vi "Read Type.vi"(8 "error in (no error)":errorcluster, 11 "VoiceMeeterRemote in":refnum<class "VoiceMeeterRemote.lvclass">) -> (0 "error out":errorcluster, 3 "VoiceMeeterRemote out":refnum<class "VoiceMeeterRemote.lvclass">)   [LabVIEW 2020, in "VoiceMeeterRemote.lvlib" / "VoiceMeeterRemote.lvclass"]
uses:
  VoiceMeeterRemote.lvclass
  VoiceMeeterRemote.lvclass/VoiceMeeterRemote.ctl
  Voicemeeter Type.ctl
  VoiceMeeterRemote.lvlib
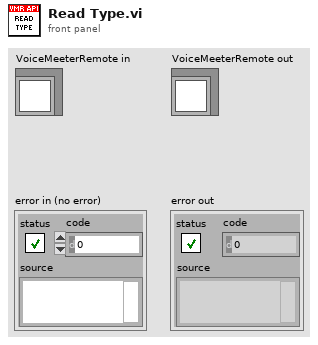
[diagram p1: front panel]
types:
  T1 = typedef "VoiceMeeterRemote.lvlib/Voicemeeter Type.ctl" = enum16{"Unknown", "Voicemeeter", "Banana", "Potato", "Potato x64"}
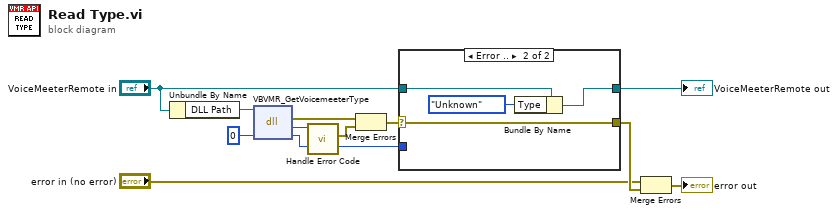
[diagram p0: block diagram]
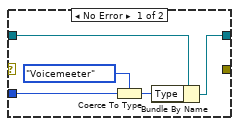
[diagram p2: hidden frame]
diagram:
  n1 = Unbundle By Name("VoiceMeeterRemote in") -> ("DLL Path"=w10:path)
  n2 = dll-call lib="C:/Program Files/National Instruments/LabVIEW 2022/user.lib/VoicemeeterRemote64/VoicemeeterRemote64.*" fn="VBVMR_GetVoicemeeterType"(path in=w10, "pType"=0) -> (error out=w7:errorcluster, "return type"=w8:i32, "pType"=w4:i32)  [unwired: 2 in, 1 out]
  n3 = call "Handle Error Code.vi"("Code"=w8) -> ("error out"=w6:errorcluster)  [unwired: 10 in]
  n4 = Merge Errors(w7, w6) -> (w5:errorcluster)
  n5 = case shown="Error .." w5 {
    selector: w5 -> [_ w21]
    tunnel: w4 -> [w17 _]
    tunnel: [_ w21] -> w12
    tunnel: "VoiceMeeterRemote in" -> [w15 w20]
    tunnel: [w13 w19] -> w1
    frame No Error {
      n6 = Coerce To Type(0:w17, 1:Voicemeeter_Type."Voicemeeter" ("Voicemeeter Type")) -> (2:w14:T1)
      n7 = Bundle By Name(cluster=w15, "Type"=w14) -> (w13:refnum<class "VoiceMeeterRemote.lvclass">)
    }
    frame Error {
      n8 = Bundle By Name(cluster=w20, "Type"=Voicemeeter_Type."Unknown") -> (w19:refnum<class "VoiceMeeterRemote.lvclass">)
    }
  }
  "VoiceMeeterRemote out" <- w1
  n9 = Merge Errors("error in (no error)", w12) -> (→"error out":errorcluster)
